vi "Get Children.vi"(8 "error in (no error)":errorcluster, 11 "NodeRef In":refnum<data-value>) -> (0 "error out":errorcluster, 2 "Children":refnum<data-value>[](array[refnum]), 3 "NodeRef":refnum<data-value>)   [LabVIEW 2020, in "PicoG-ParserLexer.lvlib" / "Node.lvclass"]
uses:
  Node.lvclass
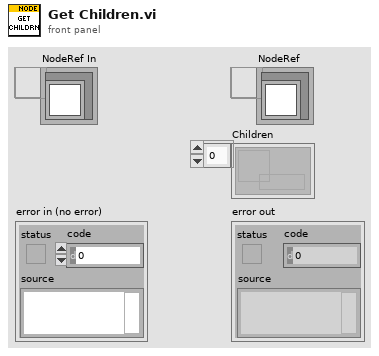
[diagram p1: front panel]
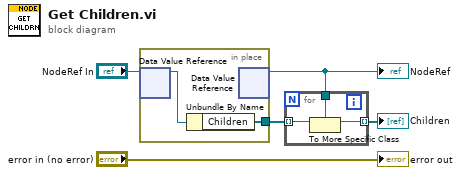
[diagram p0: block diagram]
diagram:
  n1 = in-place {
    in-place-border: [w6] -> w3
    n2 = in-place-dvr #1("NodeRef In") -> (w7:refnum<class "Node.lvclass">)  [unwired: 1 out]
    n3 = Unbundle By Name(w7) -> ("Children"=w6:refnum<data-value>[])
    n4 = in-place-dvr #1() -> (w2:refnum<data-value>)  [unwired: 1 in, 1 out]
  }
  "NodeRef" <- w2
  n5 = for {
    tunnel: [w10] -> w1 mode=indexing
    tunnel: w2 -> [w9]
    tunnel: w3 -> [w8] mode=indexing
    n6 = To More Specific Class(target class=w9, reference=w8) -> (specific class reference=w10:refnum<data-value>)  [unwired: 1 in, 1 out]
  }
  "Children" <- w1
  "error out" <- "error in (no error)"
